vi "ChirpInfo.vi"(8 "offset":i32, 11 "refnum":refnum<file>) -> (0 "% taper":sgl min=50 max=1000 format="%.2f", 1 "F2 (MHz)":sgl format="%.3f", 2 "F1 (MHz)":sgl format="%.3f", 3 "refnum out":refnum<file>, 4 "duration":sgl, 7 "Compression Parameters":T1 {"% taper" min=50 max=1000 format="%.2f"; "F2 (MHz)" format="%.3f"; "F1 (MHz)" format="%.3f"})   [LabVIEW 2022 SP3]
panel:
  out "error out":errorcluster
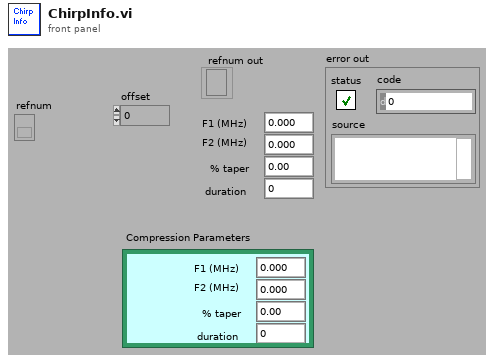
[diagram p1: front panel]
types:
  T1 = cluster{"F1 (MHz)":sgl, "F2 (MHz)":sgl, "% taper":sgl, "duration":sgl}
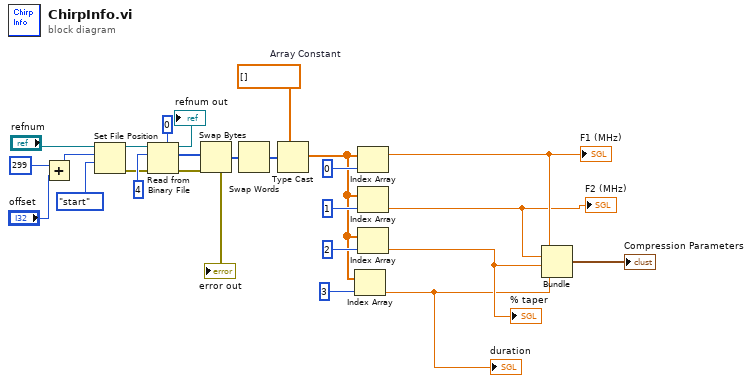
[diagram p0: block diagram]
diagram:
  w15 = sgl[] []  # Array Constant
  n1 = Add(x=299 ("pos offset (0)"), y="offset") -> (x+y=w13:i32)
  n2 = Set File Position(offset (in bytes) (0)=w13, refnum="refnum", from (0:start)=enum16{"start", "end", "current"}."start" ("pos mode (0:2)")) -> (refnum out=w11:refnum<file>, error out=w10:errorcluster)  [unwired: 1 in]
  n3 = Read from Binary File(5:0, 8:w10, 10:4 ("count"), 11:w11) -> (0:→"error out":errorcluster, 2:w16:i32[], 3:→"refnum out":refnum<file>)  [unwired: 3 out]
  n4 = Swap Bytes(anything=w16) -> (byte swapped=w18:i32[])
  n5 = Swap Words(1:w18) -> (0:w17:i32[])
  n6 = Type Cast(type=w15, x=w17) -> (*(type *) &x=w8:sgl[])
  n7 = Index Array(array=w8, index=3) -> (element=w3:sgl)
  "duration" <- w3
  n8 = Index Array(array=w8, index=0) -> (element=w6:sgl)
  "F1 (MHz)" <- w6
  n9 = Index Array(array=w8, index=1) -> (element=w5:sgl)
  "F2 (MHz)" <- w5
  n10 = Index Array(array=w8, index=2) -> (element=w4:sgl)
  "% taper" <- w4
  n11 = Bundle(w6, w5, w4, w3) -> (→"Compression Parameters":cluster{sgl, sgl, sgl, sgl})  [unwired: 1 out]
